vi "Micron Optics sm130 Acquire Continuous Spectrum.vi"() -> ()   [LabVIEW 2015]
doc: "Demonstrates acquiring continuous spectral waveform for selected channel. Only one spectral waveform is displayed each time.\n\n<b>Note:</b>\nThis example is made for the instrument without channel multiplexer. Modifications will have to be made for instruments with channel multiplexer."
uses:
  Micron Optics sm130.lvlib
panel:
  in  "Sample Rate (1000 Hz)":i32=1000
  in  "Stop":bool
  out "Spectral Waveform":T1(graph)
  in  "Channel (1: Channel 1)":u8(ring)=1 items=["Channel 1"=1, "Channel 2"=2, "Channel 3"=3, "Channel 4"=4]
  in  "VISA resource name":refnum<visa-resource-name>
  # "(c) 2009 - 2012 National Instruments.  ALL RIGHTS RESERVED."
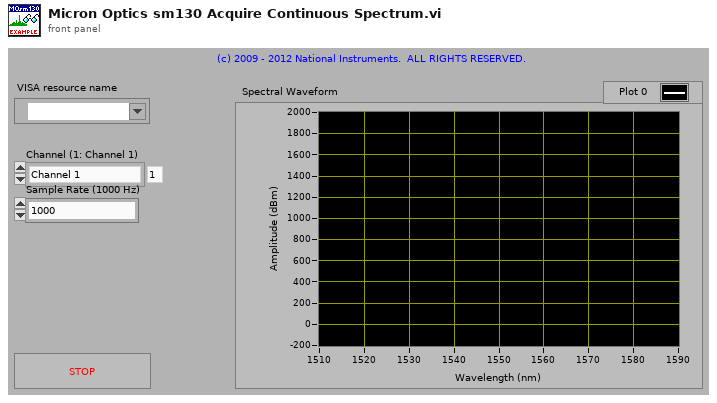
[diagram p1: front panel]
types:
  T1 = cluster{"Wavelength (nm)":dbl[], "Spectrum":i16[]}[]
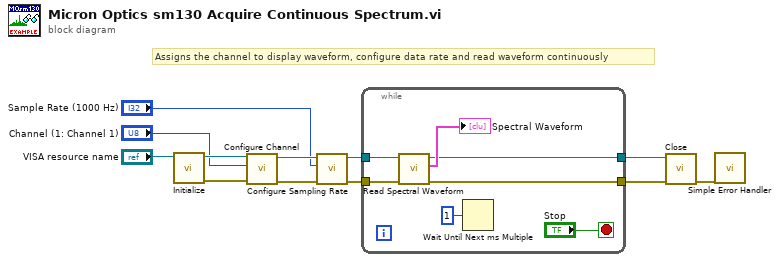
[diagram p0: block diagram]
diagram:
  # "Assigns the channel to display waveform, configure data rate and read waveform continuously"
  n1 = call "Initialize.vi"("VISA resource name"="VISA resource name") -> ("error out"=w10:errorcluster, "VISA resource name out"=w11:refnum<visa-resource-name>)  [unwired: 9 in]
  n2 = call "Configure Channel.vi"("error in (no error)"=w10, "Channel (1: Channel 1)"="Channel (1: Channel 1)", "VISA resource name"=w11) -> ("error out"=w7:errorcluster, "VISA resource name out"=w8:refnum<visa-resource-name>)  [unwired: 7 in]
  n3 = call "Configure Sampling Rate.vi"("error in (no error)"=w7, "Sample Rate (1000 Hz)"="Sample Rate (1000 Hz)", "VISA resource name"=w8) -> ("error out"=w5:errorcluster, "VISA resource name out"=w6:refnum<visa-resource-name>)  [unwired: 7 in]
  n4 = while {
    tunnel: w6 -> [w19]
    tunnel: w5 -> [w18]
    tunnel: [w16] -> w3
    tunnel: [w15] -> w2
    stop <- "Stop" stop-if-true
    n5 = call "Read Spectral Waveform.vi"("error in (no error)"=w18, "VISA resource name"=w19) -> ("error out"=w15:errorcluster, "Spectral Waveform"=→"Spectral Waveform":T1, "VISA resource name out"=w16:refnum<visa-resource-name>)  [unwired: 7 in]
    n6 = Wait Until Next ms Multiple(millisecond multiple=u32 1) -> ()  [unwired: 1 out]
  }
  n7 = call "Close.vi"("error in (no error)"=w2, "VISA resource name"=w3) -> ("error out"=w1:errorcluster)  [unwired: 9 in]
  n8 = call <vilib>:"Simple Error Handler.vi"("error in (no error)"=w1) -> ()  [unwired: 4 in, 5 out]
